vi "parse string from ADT7420 to degrees F.vi"(1 "Master Read Data String":string) -> (0 "temperature (deg F)":dbl)   [LabVIEW 8.6]
uses:
  <vilib>/express/express arith-compare/Formula/XNode/ExpressFormulaBlockNode.xnode
panel:
  out "concatenated string":string
  out "temperature (deg C)":dbl
  out "decimal":u32
  out "after substring":string
  out "before substring":string
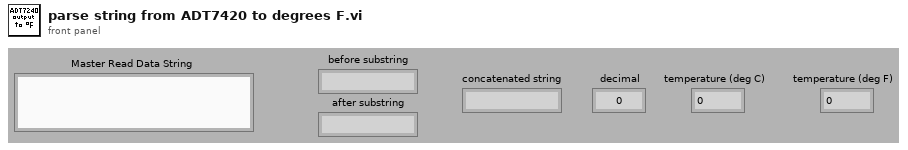
[diagram p1: front panel]
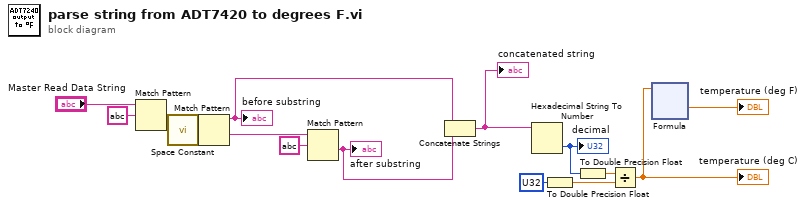
[diagram p0: block diagram]
diagram:
  n1 = Match Pattern(string="Master Read Data String", regular expression=string ?) -> (after substring=w13:string)  [unwired: 1 in, 3 out]
  n2 = call <vilib>:"Space Constant.vi"() -> ("String"=w12:string)
  n3 = Match Pattern(string=w13, regular expression=w12) -> (before substring=w9:string, after substring=w10:string)  [unwired: 1 in, 2 out]
  "before substring" <- w9
  n4 = Match Pattern(string=w10, regular expression=string ?) -> (after substring=w8:string)  [unwired: 1 in, 3 out]
  "after substring" <- w8
  n5 = Concatenate Strings(w9, w8) -> (w7:string)
  "concatenated string" <- w7
  n6 = Hexadecimal String To Number(string=w7) -> (number=w6:u32)  [unwired: 2 in, 1 out]
  "decimal" <- w6
  n7 = To Double Precision Float(number=u32 ? ("y")) -> (double precision float=w3:dbl)
  n8 = To Double Precision Float(number=w6) -> (double precision float=w4:dbl)
  n9 = Divide(x=w4, y=w3) -> (x/y=w2:dbl)
  "temperature (deg C)" <- w2
  n10 = xnode "Formula"("X1"=w2) -> ("Result"=→"temperature (deg F)":dbl)  [unwired: 1 in, 1 out]
